vi "Move Arm for Duration.vi"(6 "Synchronization":enum16{"Start", "Wait"}(ring), 7 "Description":string, 8 "Command Info In":T1, 10 "Duration (ms)":dbl, 11 "Setpoint":dbl) -> (0 "Command Info Out":T1)   [LabVIEW 2017]
doc: "This template has a parameter to control whether it waits for the command to complete or not. This is useful for operations that have a timed duration or a sensor-based duration. \n\nBe sure to right-click and select New from Template and save with a new command name."
uses:
  <vilib>/Rock Robotics/WPI/Framework/Command Status Info.ctl
  <vilib>/Rock Robotics/WPI/Framework/Completion Status.ctl
  <vilib>/Rock Robotics/WPI/Framework/Completion Notifier.ctl
  Implementation/Arm Setpoints.ctl
  Implementation/Arm Operations.ctl
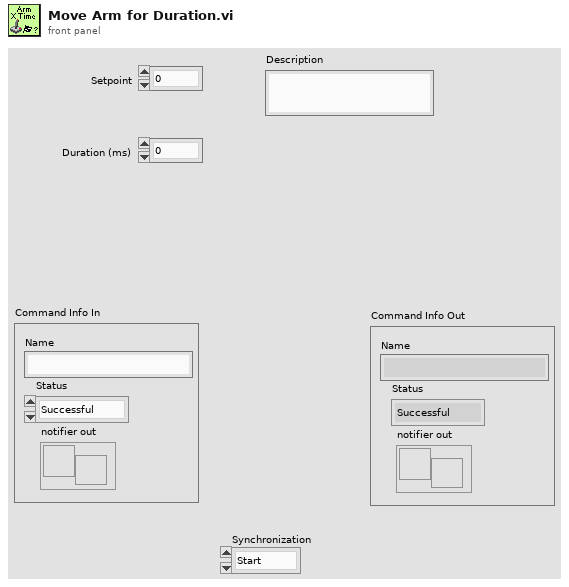
[diagram p1: front panel]
types:
  T1 = typedef "Command Status Info.ctl" = cluster{"Name":string, "Status":T2, "notifier out":T3}
  T2 = typedef "Completion Status.ctl" = enum16{"Successful", "Aborted", "Incomplete"}
  T3 = typedef "Completion Notifier.ctl" = refnum<notifier>
  T4 = typedef "Arm Setpoints.ctl" = cluster{"Operation":T5, "Setpoint":dbl, "Duration":dbl}
  T5 = typedef "Arm Operations.ctl" = enum16{"Reserve", "Read Current", "Immediate", "Move Arm for duration", "Lift Arm", "Lower Arm", "Stop Arm"}
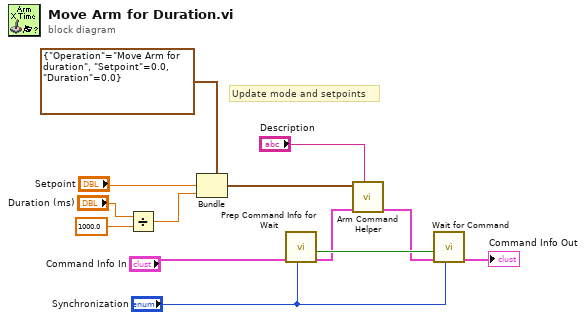
[diagram p0: block diagram]
diagram:
  # "Update mode and setpoints"
  n1 = Divide(x="Duration (ms)", y=1000.0) -> (x/y=w1:dbl)
  n2 = Bundle(cluster=T4 {"Operation"=enum."Move Arm for duration", "Setpoint"=0.0, "Duration"=0.0} ("SubSystem Data"), "Setpoint"="Setpoint", "Duration"=w1) -> (w5:T4)  [unwired: 1 in]
  n3 = call <vilib>:"Prep Command Info for Wait.vi"("Synchronication"="Synchronization", "Command Info"="Command Info In") -> ("Command Info"=w9:T1, "Allocated"=w10:bool)  [unwired: 8 in]
  n4 = call "Arm Command Helper.vi"("Description"="Description", "Command Info In"=w9, "SubSystem Data"=w5) -> ("Command Info Out"=w6:T1)  [unwired: 6 in, 2 out]
  n5 = call <vilib>:"Wait for Command.vi"("Synchronication"="Synchronization", "Command Info in"=w6, "Allocated"=w10) -> ("Command Info out"=→"Command Info Out":T1)  [unwired: 8 in]
